vi "get_MOD-Instr_devices_info.vi"(8 "error in":errorcluster) -> (0 "error out":errorcluster, 2 "device count":i32, 3 "Table":string[][](table))   [LabVIEW 2010]
uses:
  <instrlib>/niModInst/niModInst Get Installed Device Attribute (String).vi
panel:
  # "This VI queries the system information for the device names, product info, and serial \nnumber of any National Instruments product installed on your system.\n\nThis VI uses the NI-MODInst driver utility software."
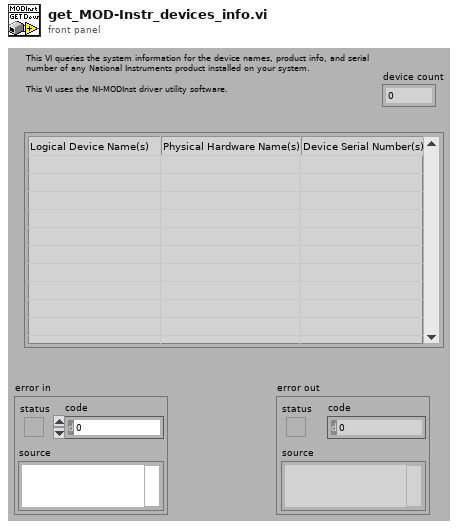
[diagram p1: front panel]
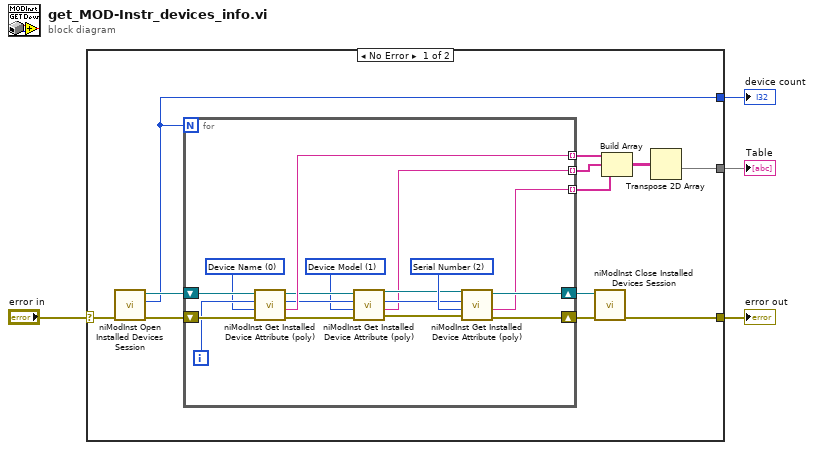
[diagram p0: block diagram]
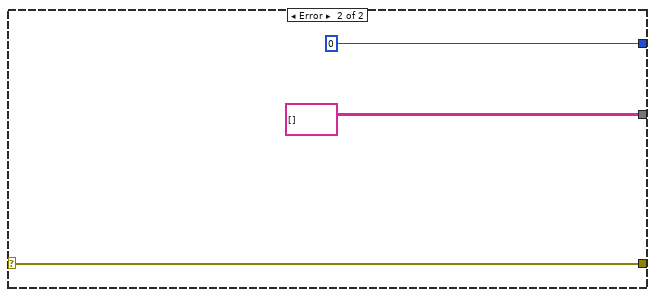
[diagram p2: hidden frame]
diagram:
  n1 = case shown="No Error" "error in" {
    selector: "error in" -> [w5 w36]
    tunnel: [w14 0 ("device count")] -> w4
    tunnel: [w7 string[][] []] -> w3
    tunnel: [w6 w36] -> w2
    frame No Error {
      n2 = call <instrlib>:"niModInst Open Installed Devices Session.vi"("error in (no error)"=w5) -> ("error out"=w16:errorcluster, "device count"=w14:i32, "session"=w15:refnum<k20>)  [unwired: 8 in]
      n3 = for {
        N: w14 -> [_]
        shift-right: [w18] -> w12
        shift-left: w15 -> [w32]
        shift-right: [w19] -> w13
        shift-left: w16 -> [w33]
        tunnel: [w29] -> w11 mode=indexing
        tunnel: [w20] -> w10 mode=indexing
        tunnel: [w17] -> w9 mode=indexing
        i -> [w31]
        w24 = 2 items=["Device Name", "Device Model", "Serial Number"] ("attribute ID")
        w25 = 1 items=["Device Name", "Device Model", "Serial Number"] ("attribute ID")
        w30 = 0 items=["Device Name", "Device Model", "Serial Number"] ("attribute ID")
        n4 = call-poly <instrlib>:"niModInst Get Installed Device Attribute (poly).vi"("error in (no error)"=w33, "attribute ID"=w30, "index in"=w31, "session in"=w32) -> ("error out"=w28:errorcluster, "attribute value"=w29:string, "index out"=w26:i32, "session out"=w27:refnum<k20>)  [unwired: 4 in]
        n5 = call-poly <instrlib>:"niModInst Get Installed Device Attribute (poly).vi"("error in (no error)"=w28, "attribute ID"=w25, "index in"=w26, "session in"=w27) -> ("error out"=w21:errorcluster, "attribute value"=w20:string, "index out"=w22:i32, "session out"=w23:refnum<k20>)  [unwired: 4 in]
        n6 = call-poly <instrlib>:"niModInst Get Installed Device Attribute (poly).vi"("error in (no error)"=w21, "attribute ID"=w24, "index in"=w22, "session in"=w23) -> ("error out"=w19:errorcluster, "attribute value"=w17:string, "session out"=w18:refnum<k20>)  [unwired: 4 in, 1 out]
      }
      n7 = call <instrlib>:"niModInst Close Installed Devices Session.vi"("error in (no error)"=w13, "session"=w12) -> ("error out"=w6:errorcluster)  [unwired: 9 in]
      n8 = Build Array(w11, w10, w9) -> (w8:string[][])
      n9 = Transpose 2D Array(2D array=w8) -> (transposed array=w7:string[][])
    }
    frame Error {
    }
  }
  "device count" <- w4
  "Table" <- w3
  "error out" <- w2
